vi "2 ControlsArbiter.vi"(11 "Prioritized Setpoint Array":T1[](array[typedef])) -> (3 "Final Setpoints":T2)   [LabVIEW 2011]
doc: "Takes in a prioritized array of clusters which contain:\n- A rudder angle setpoint and whether or not this is an override command\n- A sail position and whether or not this is an override command\n\nThe first override command encountered in the array for rudder angle and sail position (independently) defines the final setpoints. i.e. The first cluster will define the rudder angle if active rudder is True and will define the sail position if active sail is True. If one of these is not True, the algorithm will proceed to the next cluster in the array... This process repeats until the algorithm has run through the entire array."
uses:
  2 Typedefs/setpoints to boat.ctl
  2 Typedefs/sail setpt.ctl
  2 Typedefs/rudder angle.ctl
  2 Typedefs/setpoints to arbiter.ctl
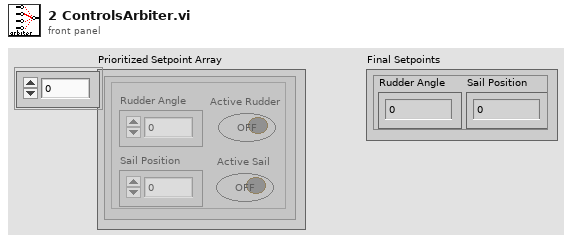
[diagram p1: front panel]
types:
  T1 = typedef "setpoints to arbiter.ctl" = cluster{"Rudder Angle":dbl, "Sail Position":dbl, "Active Rudder":bool, "Active Sail":bool}
  T2 = typedef "setpoints to boat.ctl" = cluster{"Sail Position":T3, "Rudder Angle":T4}
  T3 = typedef "sail setpt.ctl" = dbl
  T4 = typedef "rudder angle.ctl" = dbl
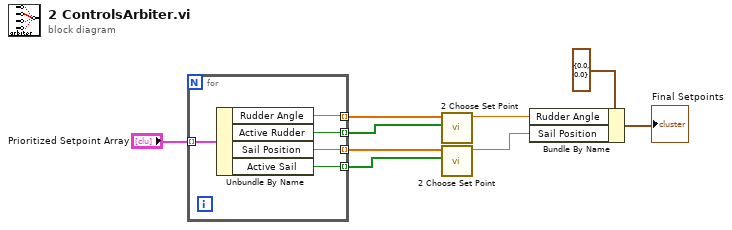
[diagram p0: block diagram]
diagram:
  n1 = for {
    tunnel: "Prioritized Setpoint Array" -> [w14] mode=indexing
    tunnel: [w13] -> w5 mode=indexing
    tunnel: [w12] -> w6 mode=indexing
    tunnel: [w11] -> w8 mode=indexing
    tunnel: [w10] -> w7 mode=indexing
    n2 = Unbundle By Name(w14) -> ("Rudder Angle"=w11:dbl, "Active Rudder"=w10:bool, "Sail Position"=w12:dbl, "Active Sail"=w13:bool)
  }
  n3 = call "2 Choose Set Point.vi"("Assert Setpoint Array"=w7, "Setpoint Array"=w8) -> ("Setpoint"=w4:dbl)  [unwired: 9 in]
  n4 = call "2 Choose Set Point.vi"("Assert Setpoint Array"=w5, "Setpoint Array"=w6) -> ("Setpoint"=w3:dbl)  [unwired: 9 in]
  n5 = Bundle By Name(cluster=T2 {"Sail Position"=0.0, "Rudder Angle"=0.0} ("Setpoints"), "Rudder Angle"=w4, "Sail Position"=w3) -> (→"Final Setpoints":T2)
